vi "Msg To Nested.vi"(8 "Alias":string, 9 "Priority?":bool, 10 "Msg":refnum<class "Msg.lvclass">, 11 "Ex Queue Actor in":refnum<class "Ex Queue Actor.lvclass">) -> (0 "error out":errorcluster)   [LabVIEW 2021, in "Ex Queue Actor.lvlib" / "Ex Queue Actor.lvclass"]
uses:
  Ex Queue Actor.lvclass
  Actor/Msg/Msg.lvclass
  Ex Queue Actor.lvclass/Ex Queue Actor.ctl
  Actor/Queue Actor/Queue Actor.lvclass
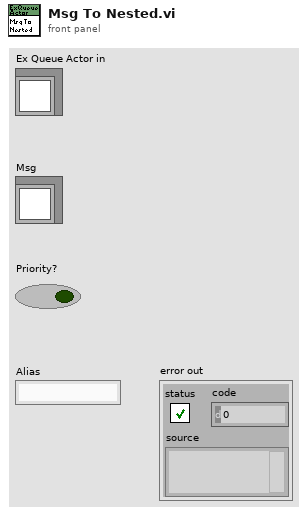
[diagram p1: front panel]
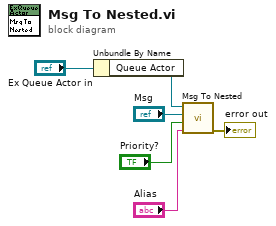
[diagram p0: block diagram]
diagram:
  n1 = Unbundle By Name("Ex Queue Actor in") -> ("Queue Actor"=w5:refnum<class "Queue Actor.lvclass">)
  n2 = call-dynamic "Msg To Nested.vi"("Alias"="Alias", "Priority?"="Priority?", "Msg"="Msg", "Queue Actor in"=w5) -> ("error out"=→"error out":errorcluster)  [unwired: 7 in]
